vi "Save_to_Project.vi"(8 "error in (no error)":errorcluster, 9 "index in":string, 10 "buildObject":T2, 11 "IB_RegData in":refnum<class "IB_RegData.lvclass">) -> (0 "error out":errorcluster, 1 "index out":string, 2 "buildObject out":T2, 3 "IB_RegData out":refnum<class "IB_RegData.lvclass">)   [LabVIEW 2020, in "IB_RegData.lvclass"]
uses:
  <vilib>/AppBuilder/IB_Classes/RegData/IB_RegData.lvclass
  <vilib>/AppBuilder/IB_Classes/RegData/IB_RegData.lvclass/IB_RegData.ctl
  <vilib>/AppBuilder/IB_RW_Project/IB_RW_Project_PropBag_Action.ctl
  <resource>/Framework/Providers/API/ItemRef.ctl
  <vilib>/AppBuilder/IB_RW_Project/IB_RW_Project_RegData_Data.ctl
panel:
  in  "data":T1
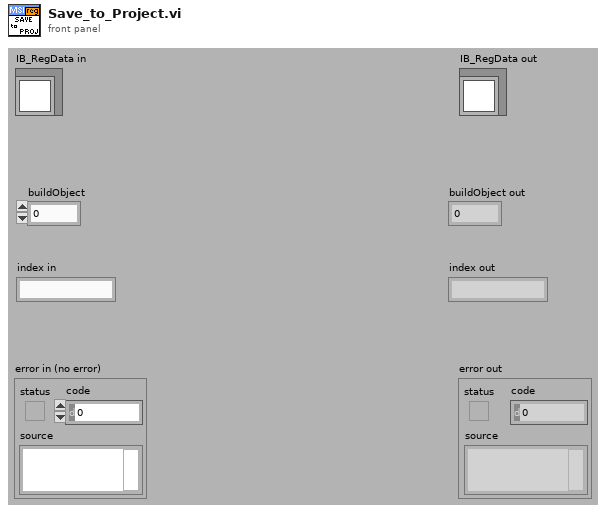
[diagram p1: front panel]
types:
  T1 = typedef "IB_RW_Project_RegData_Data.ctl" = cluster{"name":string, "unlock":bool}
  T2 = typedef "ItemRef.ctl" = u64
  T3 = typedef "IB_RW_Project_PropBag_Action.ctl" = enum16{"read", "write", "clear", "readPrevious", "writePrevious", "clearPrevious"}
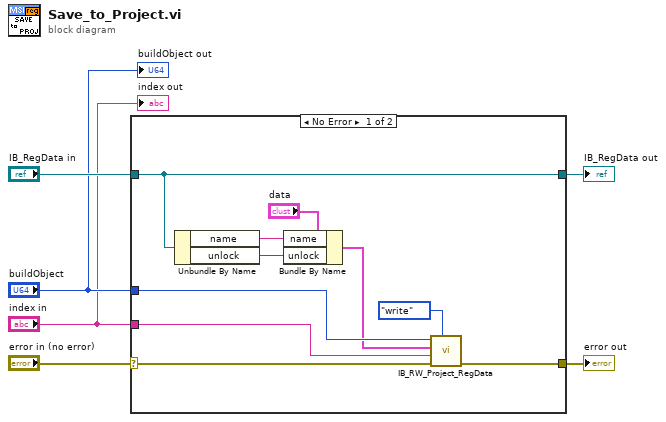
[diagram p0: block diagram]
diagram:
  n1 = case shown="No Error" "error in (no error)" {
    selector: "error in (no error)" -> [w12 w18]
    tunnel: [w11 w18] -> w5
    tunnel: [w16 w17] -> w3
    tunnel: "IB_RegData in" -> [w16 w17]
    tunnel: "buildObject" -> [w9 _]
    tunnel: "index in" -> [w8 _]
    frame No Error {
      n2 = Unbundle By Name(w16) -> ("name"=w14:string, "unlock"=w13:bool)
      n3 = Bundle By Name(cluster="data", "name"=w14, "unlock"=w13) -> (w7:T1)
      n4 = call <vilib>:"IB_RW_Project_RegData.vi"("action"=IB_RW_Project_PropBag_Action."write", "error in (no error)"=w12, "index in"=w8, "RegData"=w7, "buildObject"=w9) -> ("error out"=w11:errorcluster)  [unwired: 3 in, 3 out]
    }
    frame Error {
    }
  }
  "error out" <- w5
  "IB_RegData out" <- w3
  "buildObject out" <- "buildObject"
  "index out" <- "index in"
